vi "LEDs Loop.vi"   [LabVIEW 2016]
uses:
  <vilib>/Rock Robotics/WPI/DriverStation/WPI_DriverStationRobotMode2.ctl
  Common Code/Load State.ctl
  Common Code/Unload Mode.ctl
  Common Code/LED Indicator.ctl
  Robot Global Data.vi
  <vilib>/Rock Robotics/WPI/Solenoid/Deprecated/WPI_SolenoidSetBool.vi
types:
  T1 = typedef "Unload Mode.ctl" = enum16{"None", "Close", "Far"}
  T2 = typedef "Load State.ctl" = enum16{"Idle", "Open Flap", "Ready Close", "Ready Far"}
  T3 = typedef "WPI_DriverStationRobotMode2.ctl" = enum16{"Autonomous Disabled", "Autonomous Enabled", "Teleop Disabled", "Teleop Enabled", "Disconnected", "Finish", "Test Disabled", "Test Enabled", "Emergency Stopped"}
  T4 = typedef "Dashboard Control Data.ctl" = cluster{"Drivetrain Settings":T5, "Intake Presets ":T8, "Shooter Presets":T9, "Vision Target Packet":T10, "Auton Presets":cluster{"Start Position":dbl}, "Drivetrain Encoder Values":T11, "Drivetrain Encoder Settings":cluster{"Left Tick Constant":dbl, "Right Tick Contant":dbl, "Reset Encoders":bool, "Center Tick Constant":dbl}, "Zero Gyro":bool, "Vision Timeout":dbl, "Pressure M":dbl, "Pressure B":dbl, "Auto Agitator":T13, "Climber Settings":T14, "LEDs":T15}
  T5 = typedef "Drivetrain Settings.ctl" = cluster{"Gyro Tolerance":dbl, "Gyro Steer PID Gains":T6, "Y Power Multiplier":dbl, "Turn Power Multiplier":dbl, "Gyro Output":dbl, "Creep Rate":dbl, "Distance Drive PID Gains":T6, "Distance Tolerance":dbl, "Distance Output":dbl, "Strafe Threshold":dbl, "Strafe Correct":bool, "Strafe Tolerance":dbl, "Translate Drive PID Gains":T6, "Strafe Output":dbl, "SC Right":dbl, "SC Left":dbl, "Use Gyro":bool, "Constant Power":bool, "Strafe Power":dbl, "Input Modifier":T7, "SCR Delay":dbl, "SCL Delay":dbl}
  T6 = typedef "PID Gains.ctl" = cluster{"proportional gain (Kc)":dbl, "integral time (Ti, min)":dbl, "derivative time (Td, min)":dbl}
  T7 = typedef "Input Modifier.ctl" = enum16{"None", "Square", "Cube"}
  T8 = typedef "Intake Presets.ctl" = cluster{"Intake Speed ":dbl, "Outake Speed":dbl, "Current Trip Delay":dbl, "Max Current":dbl, "Gear Outtake Motor Delay":dbl, "Gear Intake Motor Delay":dbl, "Gear Intake Pull Up Speed":dbl, "Pusher Delay":dbl, "Release Delay":dbl, "Close Release Delay":dbl}
  T9 = typedef "Shooter Presets.ctl" = cluster{"Key Shot":cluster{"RPM ":dbl, "Hood?":bool}, "Distance Shot":cluster{"RPM":dbl, "Hood?":bool}, "RPM Tolerance":dbl, "Unstuck Delay Time ":dbl, "Initial RPM Increase":dbl, "Warmup Delay":dbl, "Faster Time":dbl, "Shooter PID Gains":cluster{"P":dbl, "I":dbl, "D":dbl, "FF":dbl, "Ramp Rate":dbl, "I Zone":dbl}, "Unstuck Trigger Power":dbl, "Trigger Power":dbl, "Unstuck RPM":dbl, "Agitator Active Power":dbl, "Agitator Idle Power":dbl, "RPM Tuning Range":dbl, "RPM M Tuning Range":dbl}
  T10 = typedef "Vision Target Packet.ctl" = cluster{"Robot Center":dbl, "Center X":dbl, "Center Y":dbl, "Angle":dbl, "Distance":dbl, "Found Target?":bool}
  T11 = typedef "Drivetrain Encoder Values.ctl" = cluster{"Left Encoder":T12, "Center Encoder":T12, "Right Encoder":T12}
  T12 = typedef "Encoder Values.ctl" = cluster{"Distance":dbl, "Speed":dbl, "Tick":dbl}
  T13 = typedef "Auto Agitator Settings.ctl" = cluster{"Enable Auto Agitation":bool, "Continuous Stir":bool, "Continuous Intake":bool, "Alternate In/Outtake":bool, "Wing Delay":dbl, "Stir Delay":dbl, "Intake Delay":dbl, "Wing On Time":dbl, "Wing Off Time":dbl, "Stir On Time":dbl, "Stir Off Time":dbl, "Intake On Time":dbl, "Intake Off Time":dbl, "Stir Power":dbl, "Intake Power":dbl, "Outtake Power":dbl, "Intake Run Time":dbl, "Outtake Run Time":dbl, "Wing$":bool, "Intake":bool, "Stirrer":bool}
  T14 = typedef "Climber Settings.ctl" = cluster{"Climber Power":dbl, "Max Current":dbl, "Avoid Current Trip?":bool}
  T15 = typedef "LED Global Data.ctl" = cluster{"Back":cluster{"Default":string, "Traction":string, "Gear Ready Close":string, "Break On":string, "Gear Loaded":string, "Climb":string, "Gear Ready Far":string, "Unload Gear":string, "Prime Unload":string}, "Front":cluster{"Default":string, "Traction":string, "Gear Ready Close":string, "Break On":string, "Gear Loaded":string, "Climb":string, "Gear Ready Far":string, "Unload Gear":string, "Prime Unload":string}, "LEDOnTime":dbl, "LEDOffTime":dbl}
  T16 = typedef "Drivetrain Command Cluster.ctl" = cluster{"Drivetrain Mode":T17, "Heading Target":dbl, "Turn Power":dbl, "Y Power":dbl, "Center Piston Down?":bool, "Traction?":bool, "Strafe Power":dbl, "Zero Gyro":bool, "Distance Target":dbl, "Strafe Correct":bool, "Y Max Output":dbl, "Y Min Output":dbl, "X Max Output":dbl, "X Min Output":dbl, "Z Max Output":dbl, "Z Min Output":dbl, "Z Target":dbl, "Brake?":bool}
  T17 = typedef "Drivetrain Mode.ctl" = enum16{"Gear Vision Align", "Manual", "Gyro Steer", "Distance Drive", "Translate Drive", "Goal Vision Align", "PID Drive"}
  T18 = typedef "Climb Command Cluster.ctl" = cluster{"Go Up":bool}
  T19 = typedef "Intake Status Cluster.ctl" = cluster{"Roller Power":dbl, "Intake Mode":T20, "Intake Auto State":T21, "Backward Tripped?":bool, "Forward Tripped?":bool, "Intake Current Trip State":T22, "Gear Flap Open":bool, "Doors Open":bool, "Traction for Gear?":bool, "Current":dbl, "Intake Down?":bool, "Gear Loaded":bool, "Pusher Activated":bool, "Gear Load State":T2, "Unload Mode":T1, "Unloading Gear?":bool}
  T20 = typedef "Intake Modes.ctl" = enum16{"Manual", "Auto"}
  T21 = typedef "Intake Auto States.ctl" = enum16{"Outtake", "Idle", "Intake", "Intake Pull Up"}
  T22 = typedef "Intake Trip States.ctl" = enum16{"Normal", "Backward Tripped", "Forward Tripped"}
  T23 = typedef "LED Indicator.ctl" = enum16{"PrimeUnload", "UnloadGear", "BrakeOn", "GearReadyClose", "GearReadyFar", "Traction", "Intake", "None", "GearIn", "Climb"}
  T24 = cluster{"Default":string, "Traction":string, "Gear Ready Close":string, "Break On":string, "Gear Loaded":string, "Climb":string, "Gear Ready Far":string, "Unload Gear":string, "Prime Unload":string}
  T25 = typedef "WPI_SolenoidDevRef.ctl" = cluster{"DevStatus":errorcluster, "Pneumatics Control Module":u8, "Forward Solenoid Channel":T26, "Reverse Solenoid Channel":T26}
  T26 = typedef "WPI_SolenoidChannel.ctl" = enum8{"Solenoid 0", "Solenoid 1", "Solenoid 2", "Solenoid 3", "Solenoid 4", "Solenoid 5", "Solenoid 6", "Solenoid 7", "Invalid"}
  T27 = typedef "LED Status Cluster.ctl" = cluster{"Front Red":bool, "Front Green":bool, "Front Blue":bool, "Back Red":bool, "Back Green":bool, "Back Blue":bool}
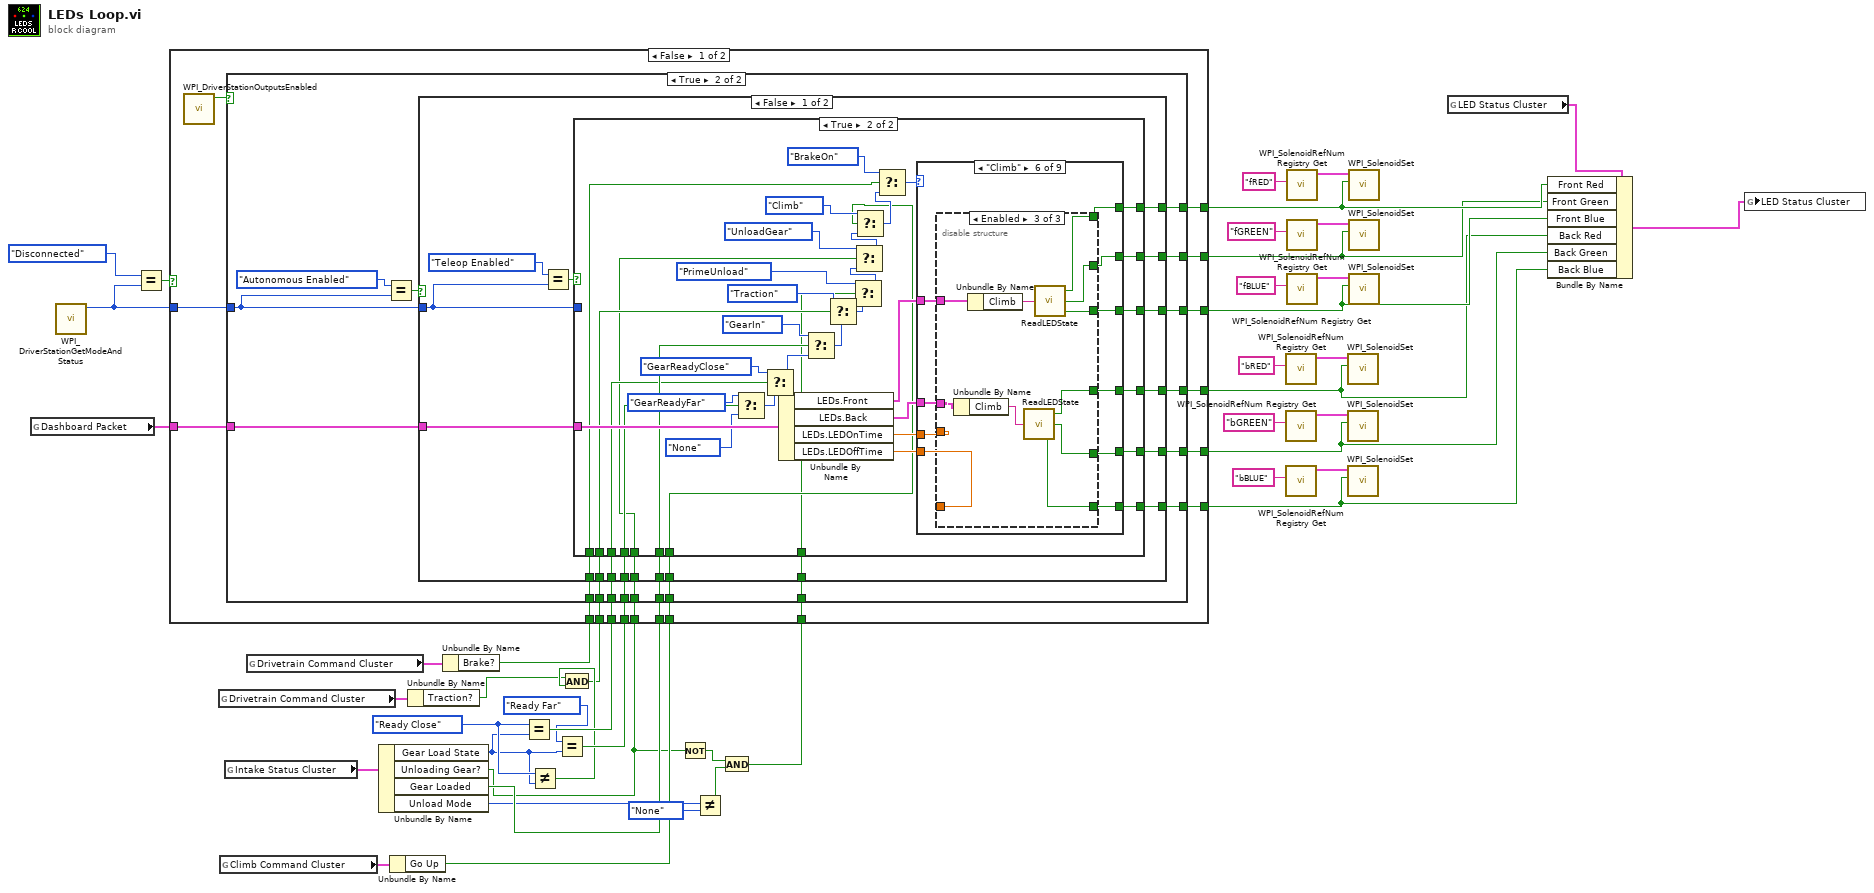
[diagram p0: block diagram]
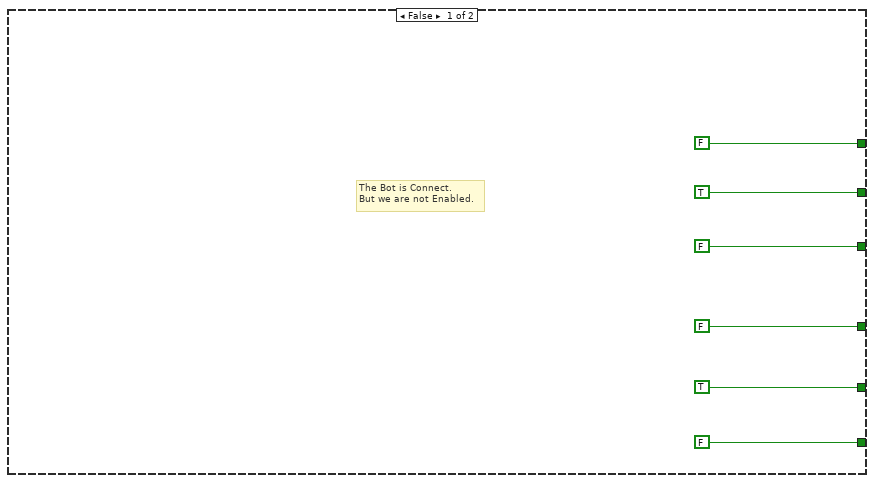
[diagram p2: hidden frame]
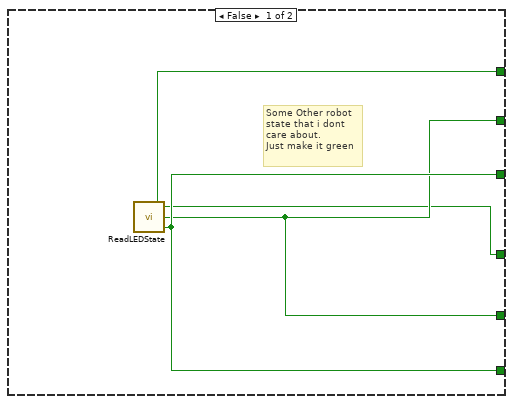
[diagram p3: hidden frame]
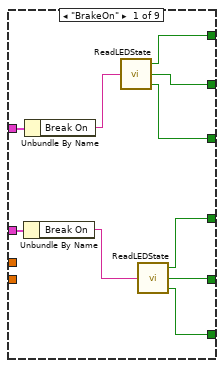
[diagram p4: hidden frame]
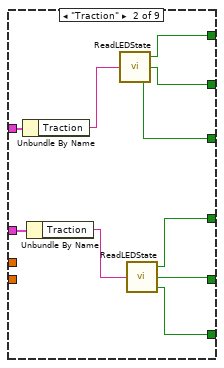
[diagram p5: hidden frame]
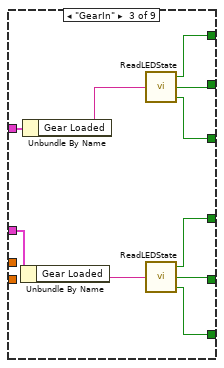
[diagram p6: hidden frame]
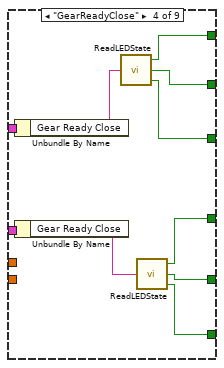
[diagram p7: hidden frame]
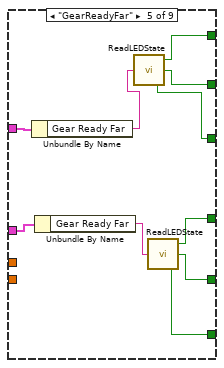
[diagram p8: hidden frame]
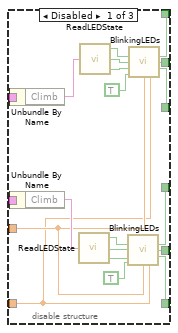
[diagram p9: hidden frame]
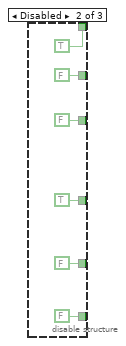
[diagram p10: hidden frame]
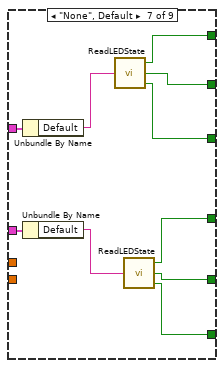
[diagram p11: hidden frame]
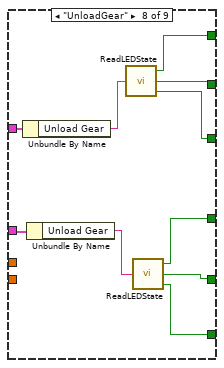
[diagram p12: hidden frame]
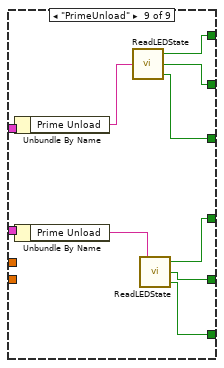
[diagram p13: hidden frame]
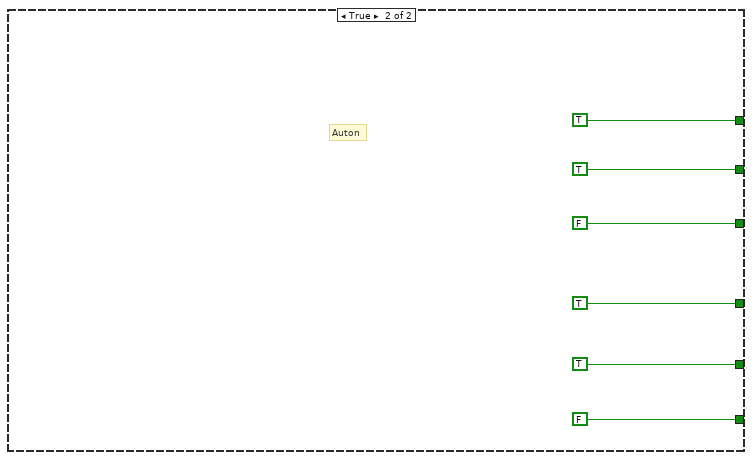
[diagram p14: hidden frame]
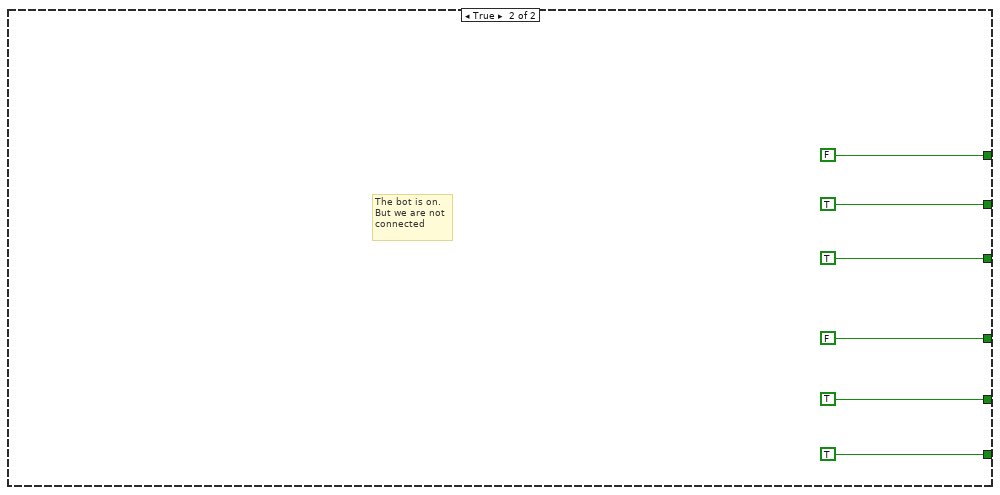
[diagram p15: hidden frame]
diagram:
  w19 = Load_State."Ready Close" ("Gear Load State")
  n1 = global read "Robot Global Data.vi" "Dashboard Packet"() -> (w27:T4)
  n2 = call <vilib>:"WPI_DriverStationGetModeAndStatus.vi"() -> ("Robot Mode"=w38:T3)  [unwired: 10 in, 1 out]
  n3 = Equal?(x=WPI_DriverStationRobotMode2."Disconnected" ("Robot Mode"), y=w38) -> (x = y?=w39:bool)
  n4 = global read "Robot Global Data.vi" "Drivetrain Command Cluster"() -> (w36:T16)
  n5 = global read "Robot Global Data.vi" "Climb Command Cluster"() -> (w24:T18)
  n6 = global read "Robot Global Data.vi" "Intake Status Cluster"() -> (w26:T19)
  n7 = global read "Robot Global Data.vi" "Drivetrain Command Cluster"() -> (w29:T16)
  n8 = Unbundle By Name(w26) -> ("Gear Load State"=w15:T2, "Unloading Gear?"=w2:bool, "Gear Loaded"=w25:bool, "Unload Mode"=w6:T1)
  n9 = Unbundle By Name(w24) -> ("Go Up"=w23:bool)
  n10 = Unbundle By Name(w36) -> ("Traction?"=w17:bool)
  n11 = Unbundle By Name(w29) -> ("Brake?"=w28:bool)
  n12 = Equal?(x=w19, y=w15) -> (x = y?=w22:bool)
  n13 = Not Equal?(x=w19, y=w15) -> (x != y?=w18:bool)
  n14 = Equal?(x=Load_State."Ready Far" ("Gear Load State"), y=w15) -> (x = y?=w20:bool)
  n15 = And(x=w17, y=w18) -> (x .and. y?=w16:bool)
  n16 = Not(x=w2) -> (.not. x?=w3:bool)
  n17 = Not Equal?(x=w6, y=Unload_Mode."None") -> (x != y?=w4:bool)
  n18 = And(x=w3, y=w4) -> (x .and. y?=w1:bool)
  n19 = case shown="False" w39 {
    tunnel: w38 -> [w61 _]
    tunnel: w28 -> [w60 _]
    tunnel: [w59 TRUE] -> w10
    tunnel: [w58 TRUE] -> w11
    tunnel: [w57 FALSE] -> w12
    tunnel: [w56 TRUE] -> w7
    tunnel: [w55 TRUE] -> w8
    tunnel: [w54 FALSE] -> w9
    tunnel: w27 -> [w53 _]
    tunnel: w25 -> [w52 _]
    tunnel: w16 -> [w51 _]
    tunnel: w23 -> [w50 _]
    tunnel: w22 -> [w49 _]
    tunnel: w20 -> [w48 _]
    tunnel: w2 -> [w47 _]
    tunnel: w1 -> [w46 _]
    frame False {
      n20 = call <vilib>:"WPI_DriverStationOutputsEnabled.vi"() -> ("OutputsEnabled?"=w62:bool)  [unwired: 10 in, 1 out]
      n21 = case shown="True" w62 {
        tunnel: w61 -> [_ w84]
        tunnel: w60 -> [_ w83]
        tunnel: [FALSE w82] -> w59
        tunnel: [TRUE w81] -> w58
        tunnel: [FALSE w80] -> w57
        tunnel: [FALSE w79] -> w56
        tunnel: [TRUE w78] -> w55
        tunnel: [FALSE w77] -> w54
        tunnel: w53 -> [_ w76]
        tunnel: w52 -> [_ w75]
        tunnel: w51 -> [_ w74]
        tunnel: w50 -> [_ w73]
        tunnel: w49 -> [_ w72]
        tunnel: w48 -> [_ w71]
        tunnel: w47 -> [_ w70]
        tunnel: w46 -> [_ w69]
        frame False {
          # "The Bot is Connect.\nBut we are not Enabled."
        }
        frame True {
          n22 = Equal?(x=WPI_DriverStationRobotMode2."Autonomous Enabled" ("Robot Mode"), y=w84) -> (x = y?=w85:bool)
          n23 = case shown="False" w85 {
            tunnel: w84 -> [w102 _]
            tunnel: w83 -> [w101 _]
            tunnel: [w100 FALSE] -> w82
            tunnel: [w99 TRUE] -> w81
            tunnel: [w98 TRUE] -> w80
            tunnel: [w97 FALSE] -> w79
            tunnel: [w96 TRUE] -> w78
            tunnel: [w95 TRUE] -> w77
            tunnel: w76 -> [w94 _]
            tunnel: w75 -> [w93 _]
            tunnel: w74 -> [w92 _]
            tunnel: w73 -> [w91 _]
            tunnel: w72 -> [w90 _]
            tunnel: w71 -> [w89 _]
            tunnel: w70 -> [w88 _]
            tunnel: w69 -> [w87 _]
            frame False {
              n24 = Equal?(x=WPI_DriverStationRobotMode2."Teleop Enabled" ("Robot Mode"), y=w102) -> (x = y?=w103:bool)
              n25 = case shown="True" w103 {
                tunnel: w102 -> [_ _]
                tunnel: w101 -> [_ w129]
                tunnel: [w107 w141] -> w100
                tunnel: [w106 w140] -> w99
                tunnel: [w105 w139] -> w98
                tunnel: [w107 w134] -> w97
                tunnel: [w106 w135] -> w96
                tunnel: [w105 w136] -> w95
                tunnel: w94 -> [_ w133]
                tunnel: w93 -> [_ w127]
                tunnel: w92 -> [_ w128]
                tunnel: w91 -> [_ w112]
                tunnel: w90 -> [_ w121]
                tunnel: w89 -> [_ w120]
                tunnel: w88 -> [_ w118]
                tunnel: w87 -> [_ w108]
                frame False {
                  # "Some Other robot\nstate that i dont\ncare about.\nJust make it green"
                  n26 = call "ReadLEDState.vi"() -> ("BLUE"=w107:bool, "GREEN"=w106:bool, "RED"=w105:bool)  [unwired: 3 in]
                }
                frame True {
                  n27 = Select(t=LED_Indicator."GearReadyFar" ("Enum"), s=w120, f=LED_Indicator."None" ("Enum")) -> (s? t:f=w123:T23)
                  n28 = Select(t=LED_Indicator."GearReadyClose" ("Enum"), s=w121, f=w123) -> (s? t:f=w130:T23)
                  n29 = Unbundle By Name(w133) -> ("LEDs.Front"=w132:T24, "LEDs.Back"=w131:T24, "LEDs.LEDOnTime"=w126:dbl, "LEDs.LEDOffTime"=w125:dbl)
                  n30 = Select(t=LED_Indicator."GearIn" ("Enum"), s=w127, f=w130) -> (s? t:f=w119:T23)
                  n31 = Select(t=LED_Indicator."Traction" ("Enum"), s=w128, f=w119) -> (s? t:f=w111:T23)
                  n32 = Select(t=LED_Indicator."PrimeUnload" ("Enum"), s=w108, f=w111) -> (s? t:f=w110:T23)
                  n33 = Select(t=LED_Indicator."UnloadGear" ("Enum"), s=w118, f=w110) -> (s? t:f=w115:T23)
                  n34 = Select(t=LED_Indicator."Climb" ("Enum"), s=w112, f=w115) -> (s? t:f=w113:T23)
                  n35 = Select(t=LED_Indicator."BrakeOn" ("Enum"), s=w129, f=w113) -> (s? t:f=w142:T23)
                  n36 = case shown="\"Climb\"" w142 {
                    tunnel: [w153 w161 w171 w183 w187 w199 w249 w253 w263] -> w141
                    tunnel: [w152 w162 w173 w182 w188 w200 w248 w254 w264] -> w140
                    tunnel: [w151 w163 w172 w181 w189 w201 w247 w255 w265] -> w139
                    tunnel: [w150 w159 w169 w180 w186 w198 w246 w252 w262] -> w136
                    tunnel: [w149 w160 w170 w179 w185 w197 w245 w251 w261] -> w135
                    tunnel: [w148 w158 w168 w178 w184 w196 w244 w250 w260] -> w134
                    tunnel: w132 -> [w147 w157 w167 w177 w193 w202 w243 w258 w268]
                    tunnel: w131 -> [w145 w155 w166 w175 w192 w203 w241 w259 w269]
                    tunnel: w126 -> [_ _ _ _ _ w195 _ _ _]
                    tunnel: w125 -> [_ _ _ _ _ w194 _ _ _]
                    frame "BrakeOn" {
                      n37 = Unbundle By Name(w145) -> ("Break On"=w144:string)
                      n38 = Unbundle By Name(w147) -> ("Break On"=w146:string)
                      n39 = call "ReadLEDState.vi"("String"=w146) -> ("BLUE"=w153:bool, "GREEN"=w152:bool, "RED"=w151:bool)  [unwired: 2 in]
                      n40 = call "ReadLEDState.vi"("String"=w144) -> ("BLUE"=w148:bool, "GREEN"=w149:bool, "RED"=w150:bool)  [unwired: 2 in]
                    }
                    frame "Traction" {
                      n41 = Unbundle By Name(w157) -> ("Traction"=w156:string)
                      n42 = Unbundle By Name(w155) -> ("Traction"=w154:string)
                      n43 = call "ReadLEDState.vi"("String"=w156) -> ("BLUE"=w161:bool, "GREEN"=w162:bool, "RED"=w163:bool)  [unwired: 2 in]
                      n44 = call "ReadLEDState.vi"("String"=w154) -> ("BLUE"=w158:bool, "GREEN"=w160:bool, "RED"=w159:bool)  [unwired: 2 in]
                    }
                    frame "GearIn" {
                      n45 = Unbundle By Name(w166) -> ("Gear Loaded"=w165:string)
                      n46 = Unbundle By Name(w167) -> ("Gear Loaded"=w164:string)
                      n47 = call "ReadLEDState.vi"("String"=w164) -> ("BLUE"=w171:bool, "GREEN"=w173:bool, "RED"=w172:bool)  [unwired: 2 in]
                      n48 = call "ReadLEDState.vi"("String"=w165) -> ("BLUE"=w168:bool, "GREEN"=w170:bool, "RED"=w169:bool)  [unwired: 2 in]
                    }
                    frame "GearReadyClose" {
                      n49 = Unbundle By Name(w177) -> ("Gear Ready Close"=w176:string)
                      n50 = Unbundle By Name(w175) -> ("Gear Ready Close"=w174:string)
                      n51 = call "ReadLEDState.vi"("String"=w176) -> ("BLUE"=w183:bool, "GREEN"=w182:bool, "RED"=w181:bool)  [unwired: 2 in]
                      n52 = call "ReadLEDState.vi"("String"=w174) -> ("BLUE"=w178:bool, "GREEN"=w179:bool, "RED"=w180:bool)  [unwired: 2 in]
                    }
                    frame "GearReadyFar" {
                      n53 = Unbundle By Name(w193) -> ("Gear Ready Far"=w191:string)
                      n54 = Unbundle By Name(w192) -> ("Gear Ready Far"=w190:string)
                      n55 = call "ReadLEDState.vi"("String"=w191) -> ("BLUE"=w187:bool, "GREEN"=w188:bool, "RED"=w189:bool)  [unwired: 2 in]
                      n56 = call "ReadLEDState.vi"("String"=w190) -> ("BLUE"=w184:bool, "GREEN"=w185:bool, "RED"=w186:bool)  [unwired: 2 in]
                    }
                    frame "Climb" {
                      n57 = disable-structure shown="Enabled" {
                        disable-tunnel: w203 -> [w223 _ w239]
                        disable-tunnel: w202 -> [w222 _ w238]
                        disable-tunnel: [w216 TRUE ("RED") w233] -> w201
                        disable-tunnel: [w215 FALSE ("GREEN") w232] -> w200
                        disable-tunnel: [w214 FALSE ("BLUE") w231] -> w199
                        disable-tunnel: [w210 TRUE ("RED") w236] -> w198
                        disable-tunnel: [w209 FALSE ("GREEN") w235] -> w197
                        disable-tunnel: [w208 FALSE ("BLUE") w234] -> w196
                        disable-tunnel: w195 -> [w205 _ _]
                        disable-tunnel: w194 -> [w204 _ _]
                        frame Disabled {
                          n58 = Unbundle By Name(w222) -> ("Climb"=w221:string)
                          n59 = Unbundle By Name(w223) -> ("Climb"=w220:string)
                          n60 = call "ReadLEDState.vi"("String"=w220) -> ("BLUE"=w213:bool, "GREEN"=w212:bool, "RED"=w211:bool)  [unwired: 2 in]
                          n61 = call "ReadLEDState.vi"("String"=w221) -> ("BLUE"=w219:bool, "GREEN"=w218:bool, "RED"=w217:bool)  [unwired: 2 in]
                          n62 = call "BlinkingLEDs.vi"("Off Time"=w204, "On Time"=w205, "RED"=w211, "GREEN"=w212, "BLUE"=w213, "Enable?"=TRUE) -> ("RED"=w210:bool, "GREEN"=w209:bool, "BLUE"=w208:bool)  [unwired: 7 in]
                          n63 = call "BlinkingLEDs.vi"("Off Time"=w204, "On Time"=w205, "RED"=w217, "GREEN"=w218, "BLUE"=w219, "Enable?"=TRUE) -> ("RED"=w216:bool, "GREEN"=w215:bool, "BLUE"=w214:bool)  [unwired: 7 in]
                        }
                        frame Disabled {
                        }
                        frame Enabled {
                          n64 = Unbundle By Name(w239) -> ("Climb"=w237:string)
                          n65 = Unbundle By Name(w238) -> ("Climb"=w230:string)
                          n66 = call "ReadLEDState.vi"("String"=w237) -> ("BLUE"=w234:bool, "GREEN"=w235:bool, "RED"=w236:bool)  [unwired: 2 in]
                          n67 = call "ReadLEDState.vi"("String"=w230) -> ("BLUE"=w231:bool, "GREEN"=w232:bool, "RED"=w233:bool)  [unwired: 2 in]
                        }
                      }
                    }
                    frame "None", Default {
                      n68 = Unbundle By Name(w243) -> ("Default"=w242:string)
                      n69 = Unbundle By Name(w241) -> ("Default"=w240:string)
                      n70 = call "ReadLEDState.vi"("String"=w242) -> ("BLUE"=w249:bool, "GREEN"=w248:bool, "RED"=w247:bool)  [unwired: 2 in]
                      n71 = call "ReadLEDState.vi"("String"=w240) -> ("BLUE"=w244:bool, "GREEN"=w245:bool, "RED"=w246:bool)  [unwired: 2 in]
                    }
                    frame "UnloadGear" {
                      n72 = Unbundle By Name(w258) -> ("Unload Gear"=w256:string)
                      n73 = Unbundle By Name(w259) -> ("Unload Gear"=w257:string)
                      n74 = call "ReadLEDState.vi"("String"=w256) -> ("BLUE"=w253:bool, "GREEN"=w254:bool, "RED"=w255:bool)  [unwired: 2 in]
                      n75 = call "ReadLEDState.vi"("String"=w257) -> ("BLUE"=w250:bool, "GREEN"=w251:bool, "RED"=w252:bool)  [unwired: 2 in]
                    }
                    frame "PrimeUnload" {
                      n76 = Unbundle By Name(w268) -> ("Prime Unload"=w267:string)
                      n77 = Unbundle By Name(w269) -> ("Prime Unload"=w266:string)
                      n78 = call "ReadLEDState.vi"("String"=w267) -> ("BLUE"=w263:bool, "GREEN"=w264:bool, "RED"=w265:bool)  [unwired: 2 in]
                      n79 = call "ReadLEDState.vi"("String"=w266) -> ("BLUE"=w260:bool, "GREEN"=w261:bool, "RED"=w262:bool)  [unwired: 2 in]
                    }
                  }
                }
              }
            }
            frame True {
              # "Auton"
            }
          }
        }
      }
    }
    frame True {
      # "The bot is on.\nBut we are not\nconnected"
    }
  }
  n80 = call <vilib>:"WPI_SolenoidRefNum Registry Get.vi"("refnum name"="bRED") -> ("SolenoidDevRef"=w30:T25)  [unwired: 9 in, 1 out]
  n81 = call <vilib>:"WPI_SolenoidRefNum Registry Get.vi"("refnum name"="bGREEN") -> ("SolenoidDevRef"=w33:T25)  [unwired: 9 in, 1 out]
  n82 = call <vilib>:"WPI_SolenoidRefNum Registry Get.vi"("refnum name"="bBLUE") -> ("SolenoidDevRef"=w34:T25)  [unwired: 9 in, 1 out]
  n83 = call <vilib>:"WPI_SolenoidRefNum Registry Get.vi"("refnum name"="fRED") -> ("SolenoidDevRef"=w45:T25)  [unwired: 9 in, 1 out]
  n84 = call <vilib>:"WPI_SolenoidRefNum Registry Get.vi"("refnum name"="fGREEN") -> ("SolenoidDevRef"=w42:T25)  [unwired: 9 in, 1 out]
  n85 = call <vilib>:"WPI_SolenoidRefNum Registry Get.vi"("refnum name"="fBLUE") -> ("SolenoidDevRef"=w41:T25)  [unwired: 9 in, 1 out]
  n86 = call-poly <vilib>:"WPI_SolenoidSet.vi"("Value"=w9, "SolenoidDevRef"=w30) -> ()  [unwired: 8 in, 2 out]
  n87 = call-poly <vilib>:"WPI_SolenoidSet.vi"("Value"=w8, "SolenoidDevRef"=w33) -> ()  [unwired: 8 in, 2 out]
  n88 = call-poly <vilib>:"WPI_SolenoidSet.vi"("Value"=w7, "SolenoidDevRef"=w34) -> ()  [unwired: 8 in, 2 out]
  n89 = call-poly <vilib>:"WPI_SolenoidSet.vi"("Value"=w12, "SolenoidDevRef"=w45) -> ()  [unwired: 8 in, 2 out]
  n90 = call-poly <vilib>:"WPI_SolenoidSet.vi"("Value"=w11, "SolenoidDevRef"=w42) -> ()  [unwired: 8 in, 2 out]
  n91 = call-poly <vilib>:"WPI_SolenoidSet.vi"("Value"=w10, "SolenoidDevRef"=w41) -> ()  [unwired: 8 in, 2 out]
  n92 = global read "Robot Global Data.vi" "LED Status Cluster"() -> (w14:T27)
  n93 = Bundle By Name(cluster=w14, "Front Red"=w12, "Front Green"=w11, "Front Blue"=w10, "Back Red"=w9, "Back Green"=w8, "Back Blue"=w7) -> (w13:T27)
  n94 = global write "Robot Global Data.vi" "LED Status Cluster"(w13) -> ()
